vi "Test.vi"() -> ()   [LabVIEW 2020]
panel:
  in  "VISA资源名称":refnum<visa-resource-name>
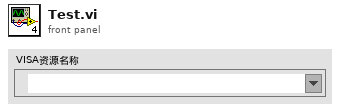
[diagram p1: front panel]
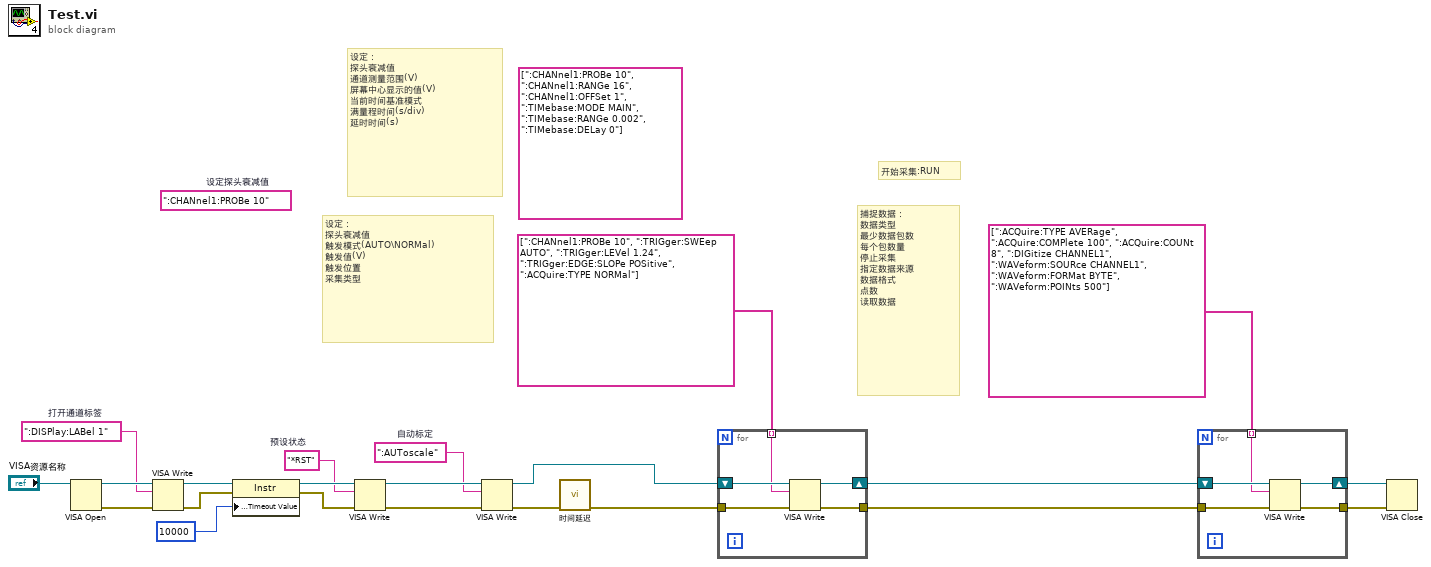
[diagram p0: block diagram]
diagram:
  (unwired) string[] [":CHANnel1:PROBe 10", ":CHANnel1:RANGe 16", ":CHANnel1:OFFSet 1", ":TIMebase:MODE MAIN", ":TIMebase:RANGe 0.002", ":TIMebase:DELay 0"]
  (unwired) ":CHANnel1:PROBe 10"  # 设定探头衰减值
  w12 = ":AUToscale"  # 自动标定
  w16 = "*RST"  # 预设状态
  w19 = ":DISPlay:LABel 1"  # 打开通道标签
  # "开始采集:RUN"
  # "捕捉数据：\n数据类型\n最少数据包数\n每个包数量\n停止采集\n指定数据来源\n数据格式\n点数\n读取数据"
  # "设定：\n探头衰减值\n触发模式(AUTO\\NORMal)\n触发值(V)\n触发位置\n采集类型"
  # "设定：\n探头衰减值\n通道测量范围(V)\n屏幕中心显示的值(V)\n当前时间基准模式\n满量程时间(s/div)\n延时时间(s)"
  n1 = VISA Open(VISA resource name="VISA资源名称") -> (VISA resource name=w20:refnum<visa-resource-name>, error out=w21:errorcluster)  [unwired: 4 in]
  n2 = VISA Write(VISA resource name=w20, write buffer=w19, error in (no error)=w21) -> (VISA resource name out=w2:refnum<visa-resource-name>, error out=w1:errorcluster)  [unwired: 1 out]
  n3 = property class="Instr"(reference=w2, error in=w1, "General Settings:Timeout Value"=u32 10000) -> (reference out=w17:refnum<visa-resource-name>, error out=w15:errorcluster)
  n4 = VISA Write(VISA resource name=w17, write buffer=w16, error in (no error)=w15) -> (VISA resource name out=w14:refnum<visa-resource-name>, error out=w13:errorcluster)  [unwired: 1 out]
  n5 = VISA Write(VISA resource name=w14, write buffer=w12, error in (no error)=w13) -> (VISA resource name out=w9:refnum<visa-resource-name>, error out=w11:errorcluster)  [unwired: 1 out]
  n6 = call "时间延迟"("error in (no error)"=w11) -> ("error out"=w10:errorcluster)  [unwired: 10 in]
  n7 = for {
    tunnel: w10 -> [w27]
    shift-right: [w25] -> w7
    shift-left: w9 -> [w26]
    tunnel: [w24] -> w6
    tunnel: string[] [":CHANnel1:PROBe 10", ":TRIGger:SWEep AUTO", ":TRIGger:LEVel 1.24", ":TRIGger:EDGE:SLOPe POSitive", ":ACQuire:TYPE NORMal"] -> [w23] mode=indexing
    n8 = VISA Write(VISA resource name=w26, write buffer=w23, error in (no error)=w27) -> (VISA resource name out=w25:refnum<visa-resource-name>, error out=w24:errorcluster)  [unwired: 1 out]
  }
  n9 = for {
    tunnel: w6 -> [w32]
    shift-right: [w30] -> w4
    shift-left: w7 -> [w31]
    tunnel: [w29] -> w3
    tunnel: string[] [":ACQuire:TYPE AVERage", ":ACQuire:COMPlete 100", ":ACQuire:COUNt 8", ":DIGitize CHANNEL1", ":WAVeform:SOURce CHANNEL1", ":WAVeform:FORMat BYTE", ":WAVeform:POINts 500"] -> [w28] mode=indexing
    n10 = VISA Write(VISA resource name=w31, write buffer=w28, error in (no error)=w32) -> (VISA resource name out=w30:refnum<visa-resource-name>, error out=w29:errorcluster)  [unwired: 1 out]
  }
  n11 = VISA Close(VISA resource name=w4, error in (no error)=w3) -> ()  [unwired: 1 out]
